vi "BoudariesToEnum.vi"(10 "max":dbl, 11 "min":dbl) -> (3 "Enum":T1)   [LabVIEW 2014]
uses:
  Enums/BoundaryStatus.ctl
  stepper3D.lvlib
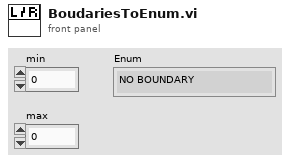
[diagram p1: front panel]
types:
  T1 = typedef "stepper3D.lvlib/BoundaryStatus.ctl" = enum16{"NO BOUNDARY", "OUT OF LEFT", "OUT OF RIGHT"}
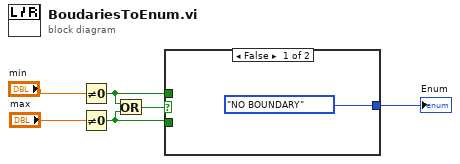
[diagram p0: block diagram]
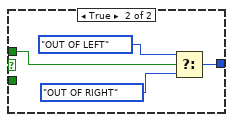
[diagram p2: hidden frame]
diagram:
  n1 = Not Equal To 0?(x="min") -> (x != 0?=w4:bool)
  n2 = Not Equal To 0?(x="max") -> (x != 0?=w5:bool)
  n3 = Or(x=w4, y=w5) -> (x .or. y?=w3:bool)
  n4 = case shown="False" w3 {
    tunnel: w4 -> [_ w11]
    tunnel: w5 -> [_ _]
    tunnel: [BoundaryStatus."NO BOUNDARY" ("Enum") w10] -> w6
    frame False {
    }
    frame True {
      n5 = Select(t=BoundaryStatus."OUT OF LEFT" ("Enum"), s=w11, f=BoundaryStatus."OUT OF RIGHT" ("Enum")) -> (s? t:f=w10:T1)
    }
  }
  "Enum" <- w6
